vi "roi custom - old.vi"(7 "Table":string[][](table), 8 "Error In":errorcluster, 9 "Cluster roi in":T1, 10 "List ROI In":dbl[][](array[numeric])=[[0.3012553778449383, 212.0, 307.0, 0.5262321564627634, 0.8298391617333317], [0.2179900662742938, 553.0, 621.0, 1.6160215122234347, 1.8333402107328942], [0.22189128311116604, 733.0, 803.0, 2.191276890630827, 2.414987315567035], [0.23707568654928451, 828.0, 903.0, 2.4948838959013955, 2.7345736369044755], [0.2412265359516473, 934.0, 1009.0, 2.8336453965190818, 3.0733351375221623], [0.2513822152119088, 1043.0, 1122.0, 3.1819944867768917, 3.4344676806334697], [0.26973683252141784, 1160.0, 1245.0, 3.5559104827416967, 3.827558855878521], [0.2678717881623769, 1262.0, 1346.0, 3.881888530505886, 4.150341040429336], [0.3655354172589007, 1993.0, 2108.0, 6.218064539482575, 6.585588809020631], [0.7506683128748562, 2149.0, 2384.0, 6.716619200768982, 7.467647055911966], [2.1181627125190436, 2011.0, 2674.0, 6.275590077323314, 8.394447387790542], [0.43800378659372247, 2675.0, 2812.0, 8.397643251003917, 8.835476511236209], [0.5591543936369769, 3248.0, 3423.0, 10.228872872267448, 10.78814893460797], [2.0749877811247526, 3255.0, 3905.0, 10.25124391476107, 12.328555003454431], [0.6538766230325155, 3874.0, 4079.0, 12.229483243839825, 12.884635202581578], [1.665395130354023, 3928.0, 4449.0, 12.402059857362042, 14.067104591530107], [2.158726430729142, 3864.0, 4539.0, 12.197524611706081, 14.354732280733803], [2.8437575673503135, 3761.0, 4651.0, 11.868350700728518, 14.712668960631735], [1.0965176651033317, 4263.0, 4606.0, 13.472674033842468, 14.568855116029887], [1.057086223423736, 4461.0, 4792.0, 14.1054549500906, 15.163285673717526], [3.6014808329940444, 4123.0, 5250.0, 13.025253183970051, 16.626991025443004], [1.8340552896834679, 4464.0, 5038.0, 14.115042539730723, 15.94946802420763], [0.8581987727342874, 5092.0, 5361.0, 16.122044637729847, 16.981731842127562], [0.7310431391128931, 5331.0, 5560.0, 16.88585594572633, 17.617708621589067], [1.0786009722571657, 5670.0, 6007.0, 17.96925357506025, 19.046259477967425], [1.4137366363648523, 5888.0, 6330.0, 18.665951755575872, 20.078523295887358], [0.9906741851963119, 7611.0, 7921.0, 24.172424072219968, 25.16314166836603]], 11 "Spectrum In":cluster{"Locations":dbl[], "Amplitudes":dbl[]}) -> (0 "Error Out":errorcluster, 2 "Cluster roi out":T1, 3 "List ROI Out":dbl[][](array[numeric]))   [LabVIEW 2020]
uses:
  <vilib>/Utility/miscctls.llb/LVRangeTypeDef.ctl
panel:
  out "subarray":dbl[](array[numeric])
  in  "Stop Button":bool
  out "Spectrum":cluster{"Locations":dbl[], "Amplitudes":dbl[]}[](graph)
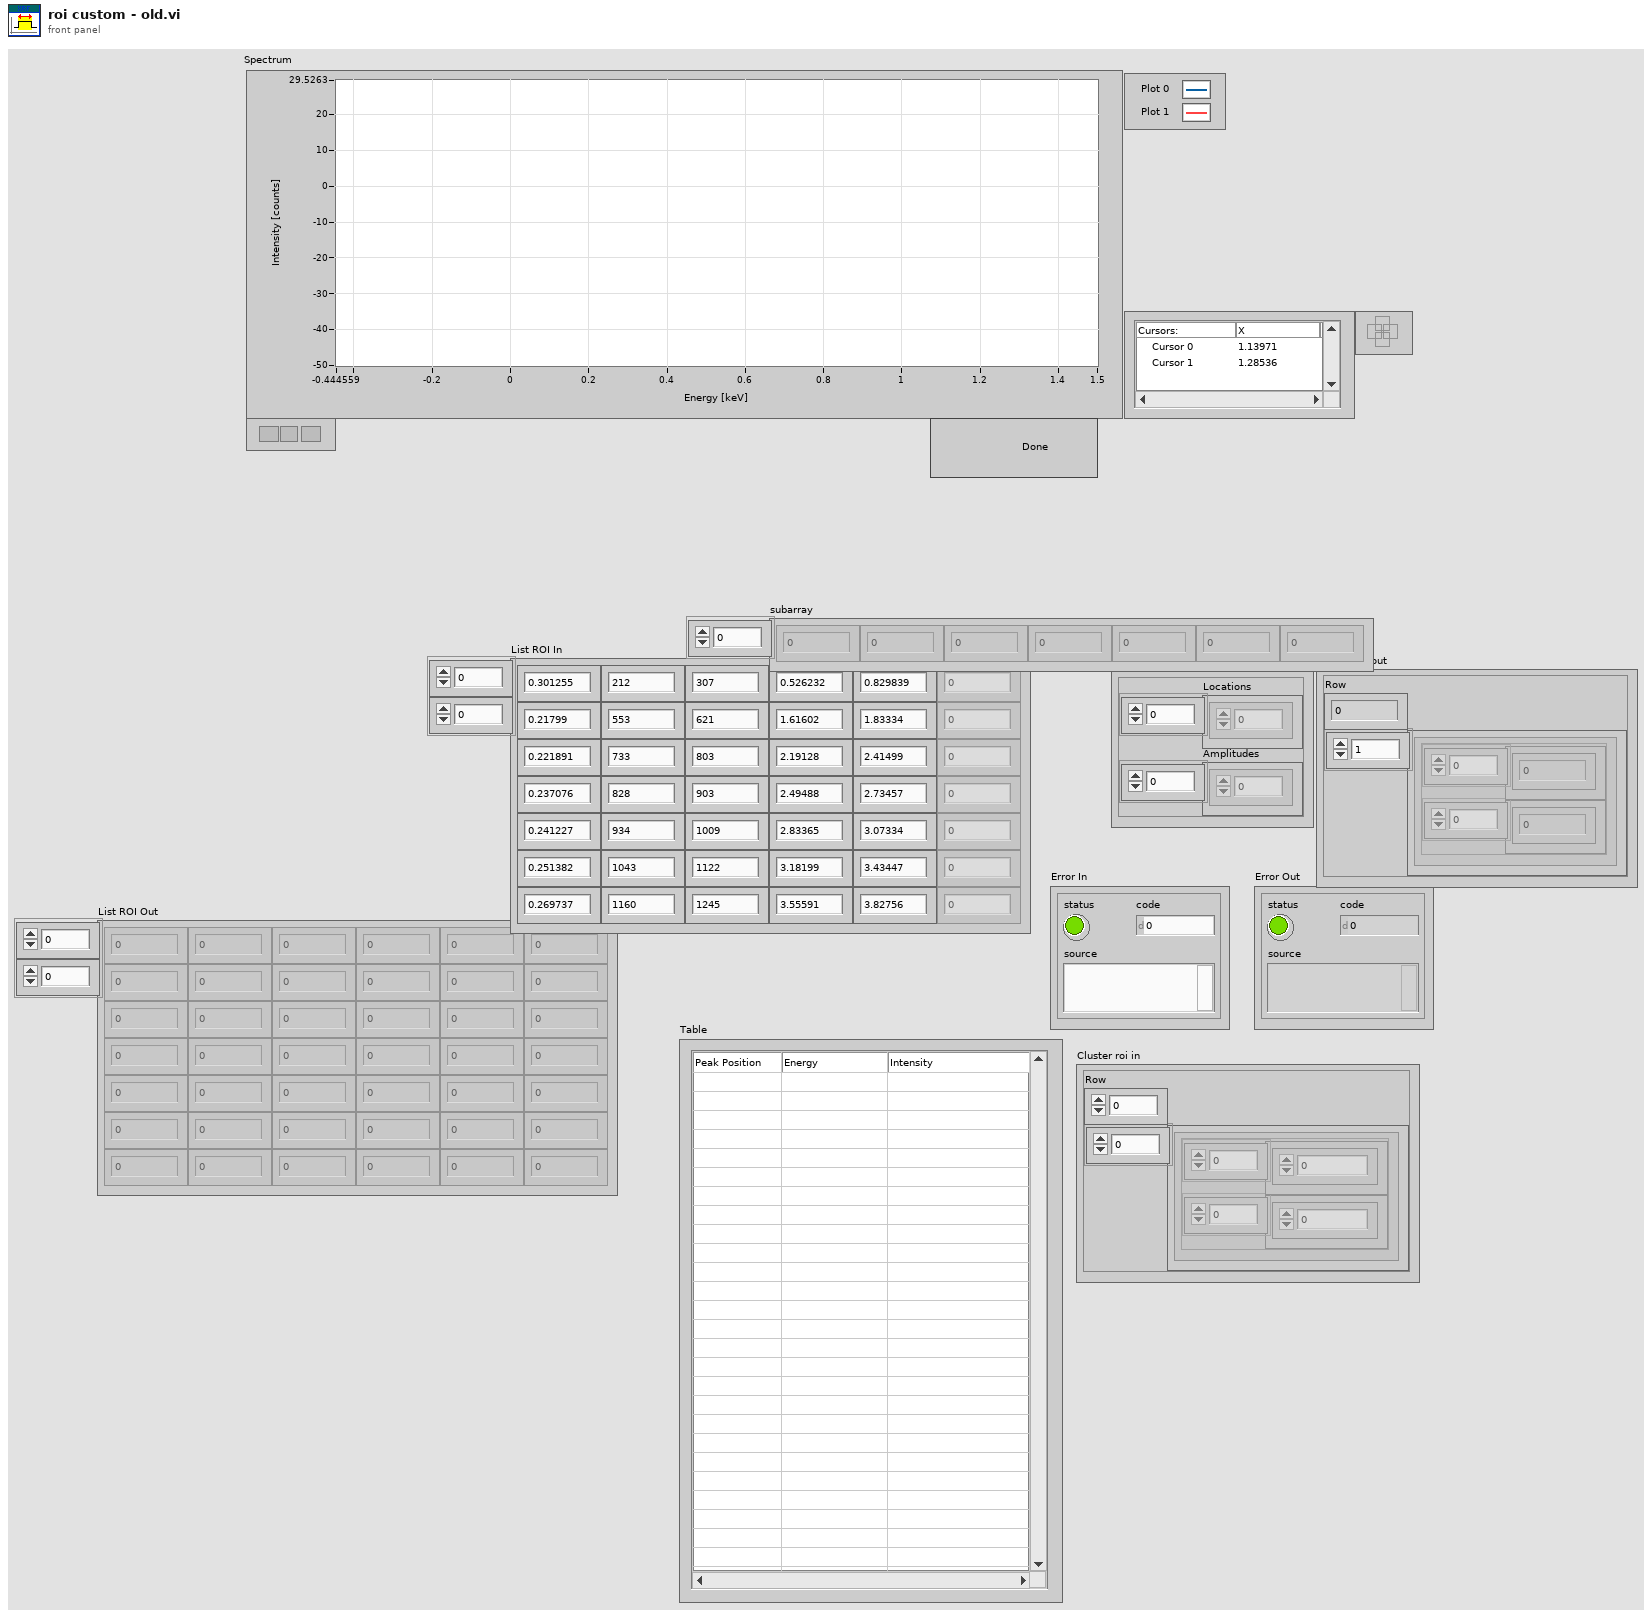
[diagram p1: front panel]
types:
  T1 = cluster{"Row":i32, "Array":cluster{"Array":dbl[], "Array":dbl[]}[]}
  T2 = cluster{"Ch0":dbl, "Ch1":dbl, "E0":dbl, "E1":dbl}
  T3 = typedef "LVRangeTypeDef.ctl" = cluster{"Minimum":dbl, "Maximum":dbl, "Increment":dbl, "Minor Increment":dbl, "Start":dbl}
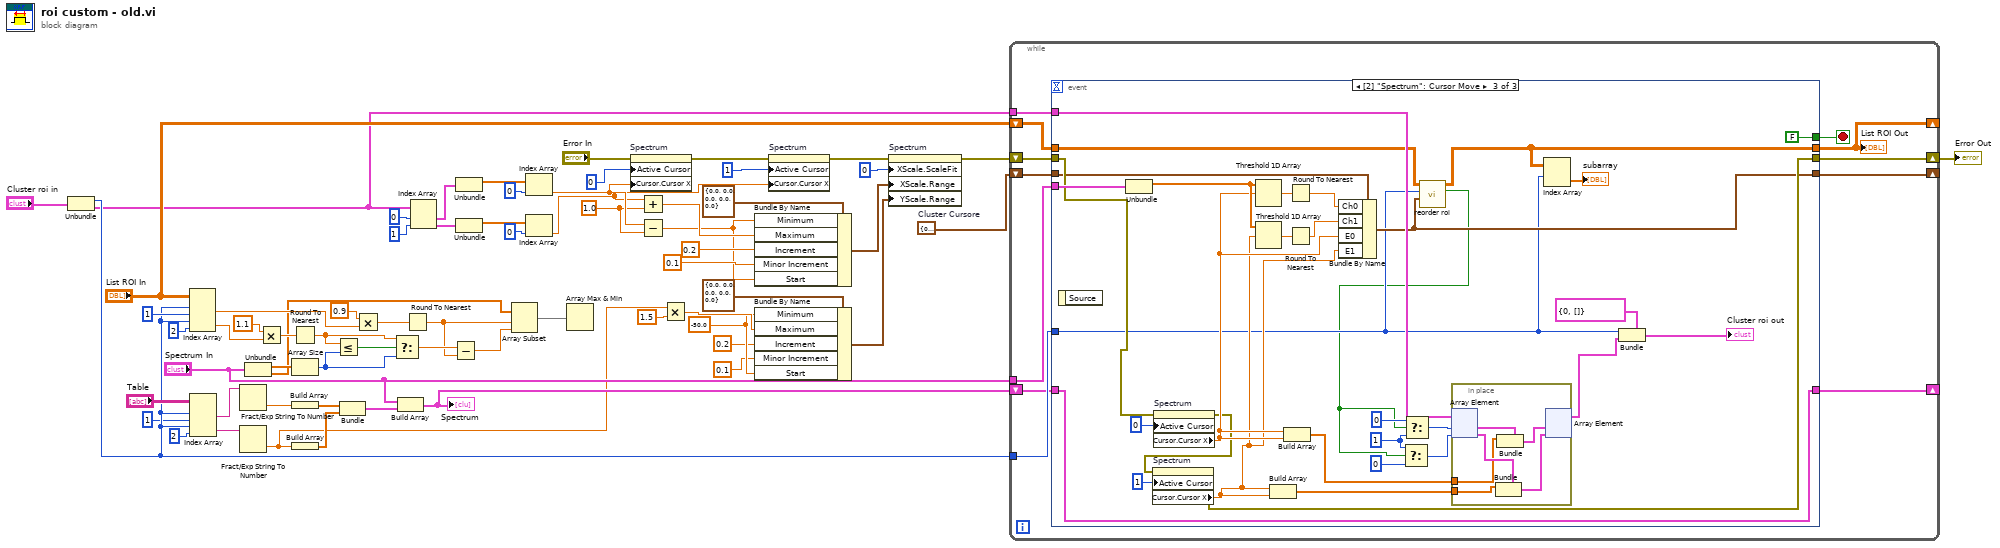
[diagram p0: block diagram]
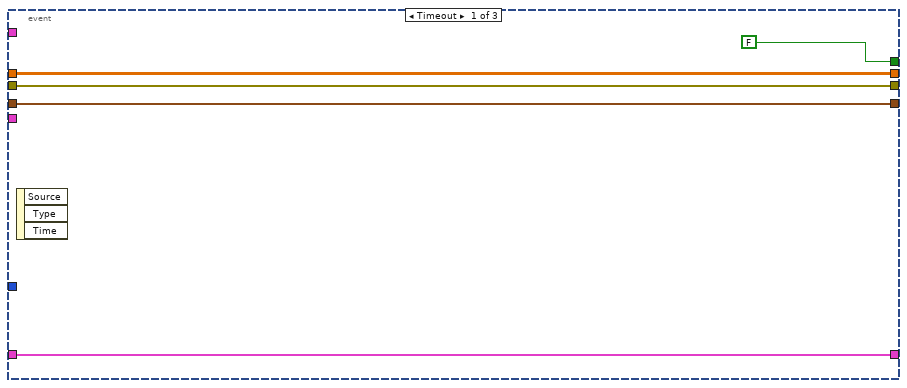
[diagram p2: hidden frame]
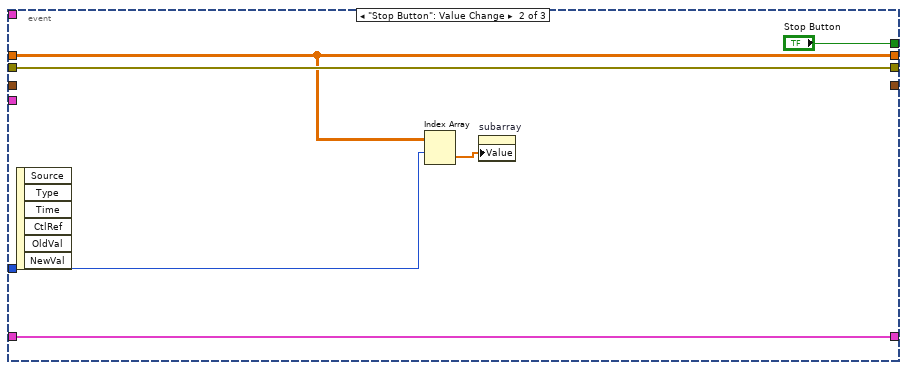
[diagram p3: hidden frame]
diagram:
  w2 = T2 {"Ch0"=0.0, "Ch1"=0.0, "E0"=0.0, "E1"=0.0}  # Cluster Cursore
  w19 = -50.0 ("Minimum")
  w48 = 1.0 ("y")
  n1 = Unbundle("Cluster roi in") -> ("Row"=w14:i32, "Array"=w4:cluster{"Array":dbl[], "Array":dbl[]}[])
  n2 = Index Array(array="List ROI In", index (row) #1=w14, index (col) #1=1 ("disabled index (col)"), index (row) #2=w14, index (col) #2=2 ("disabled index (col)")) -> (element #1=w43:dbl, element #2=w42:dbl)
  n3 = Index Array(array="Table", index (row) #1=w14, index (col) #1=1, index (row) #2=w14, index (col) #2=2) -> (element #1=w11:string, element #2=w10:string)
  n4 = Fract/Exp String To Number(string=w11) -> (number=w7:dbl)  [unwired: 3 in, 1 out]
  n5 = Fract/Exp String To Number(string=w10) -> (number=w1:dbl)  [unwired: 3 in, 1 out]
  n6 = Unbundle("Spectrum In") -> ("Locations"=w39:dbl[], "Amplitudes"=w32:dbl[])
  n7 = Multiply(x=1.1, y=w42) -> (x*y=w40:dbl)
  n8 = Round To Nearest(number=w40) -> (nearest integer value=w37:dbl)
  n9 = Array Size(array=w39) -> (size(s)=w36:i32)
  n10 = Build Array(w7) -> (w6:dbl[])
  n11 = Build Array(w1) -> (w5:dbl[])
  n12 = Less Or Equal?(x=w37, y=w36) -> (x <= y?=w38:bool)
  n13 = Bundle(w6, w5) -> (w8:cluster{dbl[], dbl[]})  [unwired: 1 in]
  n14 = Multiply(x=0.9, y=w43) -> (x*y=w41:dbl)
  n15 = Select(t=w37, s=w38, f=w36) -> (s? t:f=w35:dbl)
  n16 = Build Array("Spectrum In", w8) -> (w3:cluster{"Locations":dbl[], "Amplitudes":dbl[]}[])
  "Spectrum" <- w3
  n17 = Round To Nearest(number=w41) -> (nearest integer value=w33:dbl)
  n18 = Index Array(array=w4, index #1=0 ("index"), index #2=1 ("index")) -> (element #1=w63:cluster{"Array":dbl[], "Array":dbl[]}, element #2=w62:cluster{"Array":dbl[], "Array":dbl[]})
  n19 = Subtract(x=w35, y=w33) -> (x-y=w34:dbl)
  n20 = Unbundle(w63) -> ("Array"=w61:dbl[])  [unwired: 1 out]
  n21 = Unbundle(w62) -> ("Array"=w58:dbl[])  [unwired: 1 out]
  n22 = Array Subset(array=w32, index=w33, length=w34) -> (w28:dbl[])
  n23 = Index Array(array=w61, index=0) -> (element=w51:dbl)
  n24 = Index Array(array=w58, index=0) -> (element=w49:dbl)
  n25 = Array Max & Min(array=w28) -> ()  [unwired: 4 out]
  n26 = property on="Spectrum" class="XYGraph (strict)"(error in="Error In", "Active Cursor"=u32 0, "Cursor.Cursor X"=w51) -> (error out=w56:errorcluster)  [unwired: 1 in, 1 out]
  n27 = Add(x=w49, y=w48) -> (x+y=w50:dbl)
  n28 = Subtract(x=w51, y=w48) -> (x-y=w20:dbl)
  n29 = Multiply(x=w1, y=1.5) -> (x*y=w31:dbl)
  n30 = Bundle By Name(cluster=T3 {"Minimum"=0.0, "Maximum"=0.0, "Increment"=0.0, "Minor Increment"=0.0, "Start"=0.0} ("output cluster"), "Minimum"=w20, "Maximum"=w50, "Increment"=0.2, "Minor Increment"=0.1 ("Increment"), "Start"=w20) -> (w26:T3)
  n31 = Bundle By Name(cluster=T3 {"Minimum"=0.0, "Maximum"=0.0, "Increment"=0.0, "Minor Increment"=0.0, "Start"=0.0} ("Y Scale.Range"), "Minimum"=w19, "Maximum"=w31, "Increment"=0.2, "Minor Increment"=0.1 ("Increment"), "Start"=w19) -> (w16:T3)
  n32 = property on="Spectrum" class="XYGraph (strict)"(error in=w56, "Active Cursor"=u32 1, "Cursor.Cursor X"=w49) -> (error out=w52:errorcluster)  [unwired: 1 in, 1 out]
  n33 = property on="Spectrum" class="XYGraph (strict)"(error in=w52, "XScale.ScaleFit"=u8 0 ("X Scale.Scale Fit"), "XScale.Range"=w26, "YScale.Range"=w16) -> (error out=w23:errorcluster)  [unwired: 1 in, 1 out]
  n34 = while {
    shift-right: [w75] -> w53
    shift-left: w23 -> [w77]
    shift-right: [w72] -> _
    shift-left: "List ROI In" -> [w76]
    tunnel: "Spectrum In" -> [w74]
    tunnel: w14 -> [w73]
    tunnel: w4 -> [w71]
    shift-right: [w69] -> _
    shift-left: w3 -> [w70]
    shift-right: [w68] -> _
    shift-left: w2 -> [w67]
    stop <- w78 stop-if-true
    n35 = event shown="[2] \"Spectrum\": Cursor Move" {
      selector: _ -> [_ _ _]
      dyn-events: _ -> [_ _ _]
      timeout: _ -> [_ _ _]
      tunnel: [FALSE ("Stop Button") "Stop Button" FALSE ("Stop Button")] -> w78
      tunnel: w77 -> [w82 w88 w116]
      tunnel: [w79 w84 w92] -> w72
      tunnel: w76 -> [w79 w84 w94]
      tunnel: [w82 w88 w115] -> w75
      tunnel: w74 -> [_ _ w121]
      tunnel: w73 -> [_ w85 w91]
      tunnel: w71 -> [_ _ w105]
      tunnel: w70 -> [w81 w87 w114]
      tunnel: [w81 w87 w114] -> w69
      tunnel: [w80 _ w95] -> w68
      tunnel: w67 -> [w80 _ w106]
      event Timeout {
        n36 = event-data() -> ()  [unwired: 1 in, 3 out]
      }
      event "Stop Button": Value Change {
        n37 = event-data() -> ()  [unwired: 1 in, 6 out]
        n38 = Index Array(array=w84, index (row)=w85) -> (element=w86:dbl[])  [unwired: 1 in]
        n39 = property on="subarray" class="Arr (strict)"("Value"=w86) -> ()  [unwired: 2 in, 2 out]
      }
      event "Spectrum": Cursor Move {
        w103 = 1 ("index")
        n40 = event-data() -> ()  [unwired: 1 in, 1 out]
        n41 = Unbundle(w121) -> ("Locations"=w111:dbl[])  [unwired: 1 out]
        n42 = property on="Spectrum" class="XYGraph (strict)"(error in=w116, "Active Cursor"=u32 0) -> (error out=w99:errorcluster, "Cursor.Cursor X"=w108:dbl)  [unwired: 1 in, 1 out]
        n43 = property on="Spectrum" class="XYGraph (strict)"(error in=w99, "Active Cursor"=u32 1) -> (error out=w115:errorcluster, "Cursor.Cursor X"=w107:dbl)  [unwired: 1 in, 1 out]
        n44 = Threshold 1D Array(2:w108, 3:w111) -> (0:w113:dbl)  [unwired: 1 in]
        n45 = Threshold 1D Array(2:w107, 3:w111) -> (0:w112:dbl)  [unwired: 1 in]
        n46 = Build Array(w107, w107) -> (w97:dbl[])
        n47 = Build Array(w108, w108) -> (w98:dbl[])
        n48 = Round To Nearest(number=w113) -> (nearest integer value=w110:dbl)
        n49 = Round To Nearest(number=w112) -> (nearest integer value=w109:dbl)
        n50 = Bundle By Name(cluster=w106, "Ch0"=w110, "Ch1"=w109, "E0"=w108, "E1"=w107) -> (w95:T2)
        n51 = call "reorder roi.vi"("Cluster Cursori"=w95, "Peak"=w91, "List ROI In in"=w94) -> ("invert?"=w90:bool, "List ROI In out"=w92:dbl[][])  [unwired: 7 in]
        n52 = Select(t=w103, s=w90, f=0 ("index")) -> (s? t:f=w100:i32)
        n53 = Select(t=0 ("index"), s=w90, f=w103) -> (s? t:f=w101:i32)
        n54 = in-place {
          in-place-border: w98 -> [w124]
          in-place-border: w97 -> [w123]
          n55 = in-place-array #1(w105, w101, w100) -> (w128:cluster{"Array":dbl[], "Array":dbl[]}, w127:cluster{"Array":dbl[], "Array":dbl[]})
          n56 = Bundle(cluster=w127, "Array"=w123) -> (w125:cluster{"Array":dbl[], "Array":dbl[]})  [unwired: 1 in]
          n57 = Bundle(cluster=w128, "Array"=w124) -> (w126:cluster{"Array":dbl[], "Array":dbl[]})  [unwired: 1 in]
          n58 = in-place-array #1(w126, w125) -> (w96:cluster{"Array":dbl[], "Array":dbl[]}[])  [unwired: 2 out]
        }
        n59 = Index Array(array=w92, index (row)=w91) -> (element=→"subarray":dbl[])  [unwired: 1 in]
        n60 = Bundle(cluster=cluster{i32, cluster{dbl[], dbl[]}[]} {0, []}, w91, w96) -> (→"Cluster roi out":cluster{i32, cluster{dbl[], dbl[]}[]})
      }
    }
    "List ROI Out" <- w72
  }
  "Error Out" <- w53
